vi "userstatusRW.vi"(7 "write?":bool, 8 "username":string, 10 "status":u16, 11 "Cluster in":T1 {"mode" items=["classic", "countdown", "ai"]; "player"."status" items=["host_ready", "idle", "host", "leaved", "ready", "playing", "lose(mine)", "lose(ot)", "win"]}) -> (2 "status out":u16, 3 "Cluster out":T1 {"mode" items=["classic", "countdown", "ai"]; "player"."status" items=["host_ready", "idle", "host", "leaved", "ready", "playing", "lose(mine)", "lose(ot)", "win"]})   [LabVIEW 2025]
uses:
  controls/playerstatus.ctl
  multi.ctl
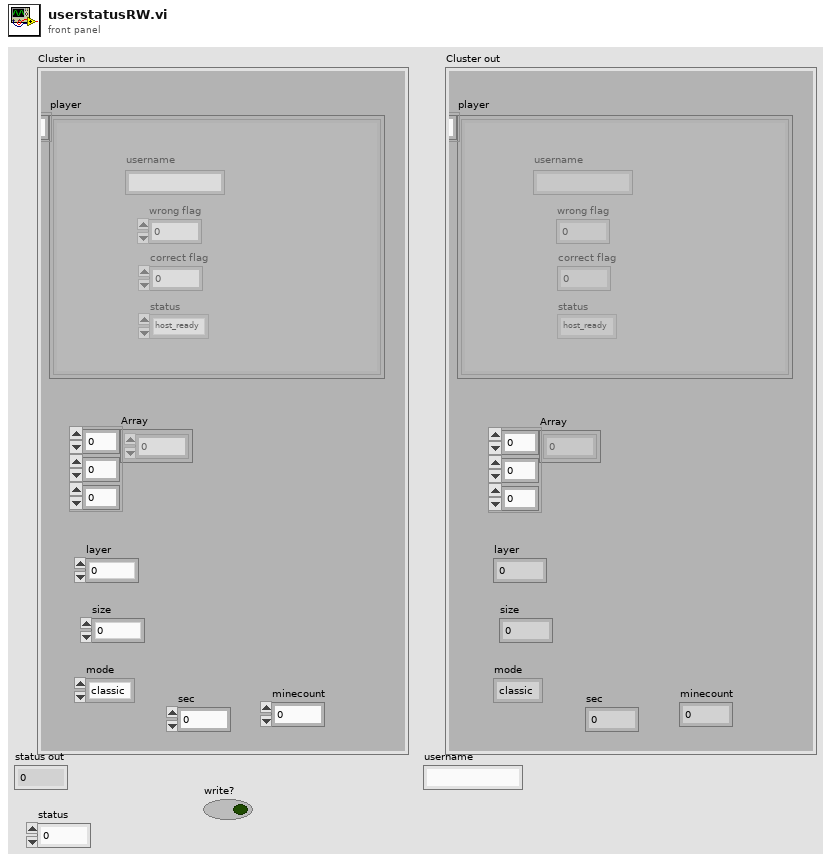
[diagram p1: front panel]
types:
  T1 = typedef "multi.ctl" = cluster{"Array":i8[][][], "player":T2[], "layer":i32, "size":i32, "mode":u16, "sec":i32, "minecount":i32}
  T2 = typedef "playerstatus.ctl" = cluster{"correct flag":i32, "wrong flag":i32, "username":string, "status":u16}
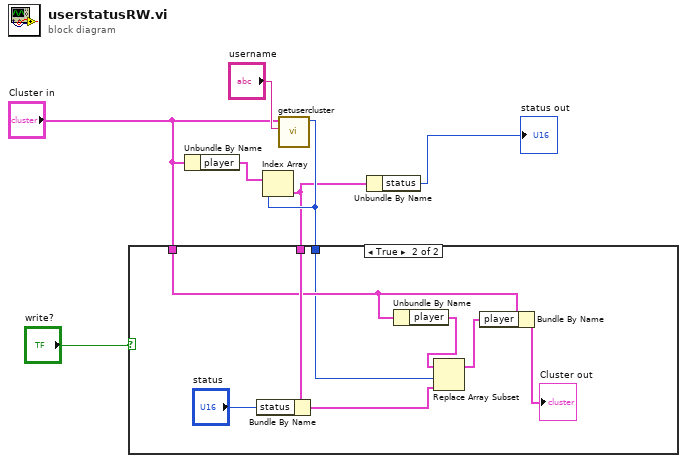
[diagram p0: block diagram]
diagram:
  n1 = Unbundle By Name("Cluster in") -> ("player"=w7:T2[])
  n2 = call "getusercluster.vi"("username"="username", "multiplayer"="Cluster in") -> ("Numeric"=w4:i32)  [unwired: 9 in]
  n3 = Index Array(array=w7, index=w4) -> (element=w3:T2)
  n4 = case shown="True" "write?" {
    tunnel: w3 -> [_ w11]
    tunnel: "Cluster in" -> [_ w9]
    tunnel: w4 -> [_ w8]
    frame False {
    }
    frame True {
      n5 = Bundle By Name(cluster=w11, "status"="status") -> (w15:T2)
      n6 = Unbundle By Name(w9) -> ("player"=w13:T2[])
      n7 = Replace Array Subset(array=w13, new element=w15, index=w8) -> (w14:T2[])
      n8 = Bundle By Name(cluster=w9, "player"=w14) -> (→"Cluster out":T1)
    }
  }
  n9 = Unbundle By Name(w3) -> ("status"=→"status out":u16)
